vi "GetFieldFromProtobufIndexniswitch_grpc_SetAttributeViInt32Request_attribute_value_enum.vi"(1 "protobuf index":i32) -> (0 "oneof field name":string)   [LabVIEW 2021, in "NI Switch_client.lvlib" / "niswitch_grpc_SetAttributeViInt32Request_attribute_value_enum.lvclass"]
uses:
  niswitch_grpc_SetAttributeViInt32Request_attribute_value_enum.lvclass
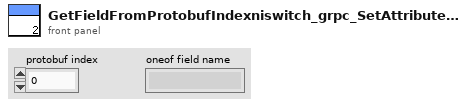
[diagram p1: front panel]
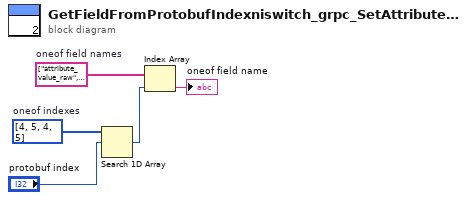
[diagram p0: block diagram]
diagram:
  w5 = string[] ["attribute_value_raw", "attribute_value", "attribute_value_raw", "attribute_value"]  # oneof field names
  w4 = i32[] [4, 5, 4, 5]  # oneof indexes
  n1 = Search 1D Array(1D array=w4, element="protobuf index") -> (index of element=w2:i32)  [unwired: 1 in]
  n2 = Index Array(array=w5, index=w2) -> (element=→"oneof field name":string)
